vi "JSON to LVObject - Offset - Skipps Previous Data.vi"() -> ()   [LabVIEW 2017, in "JSON Serializable Serializer Tests.lvlib"]
uses:
  JSON Serializable Serializer Tests.lvlib
  JSON Serializable Serializer/JSON Serializable Serializer.lvclass
  Mock JSON Serializable/Mock JSON Serializable.lvclass/Mock JSON Serializable.ctl
  <vilib>/addons/_JKI Toolkits/Caraya/classes/Assert/Assert Equal Value and Type_Variant.vi
  <vilib>/addons/_JKI Toolkits/Caraya/classes/Test/Test.lvclass
  <vilib>/addons/_JKI Toolkits/Caraya/classes/Assert/Assert.lvclass
  Mock JSON Serializable/Mock JSON Serializable.lvclass
panel:
  out "error out":errorcluster
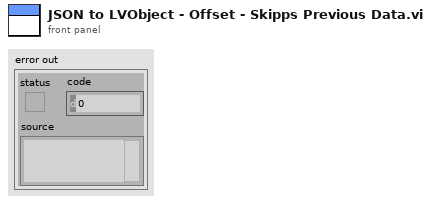
[diagram p1: front panel]
types:
  T1 = cluster{"LVClass Serializer":refnum<class "JSONtext LVClass Serializer.lvclass">, "<JSON>":string, "error in (no error)":errorcluster}
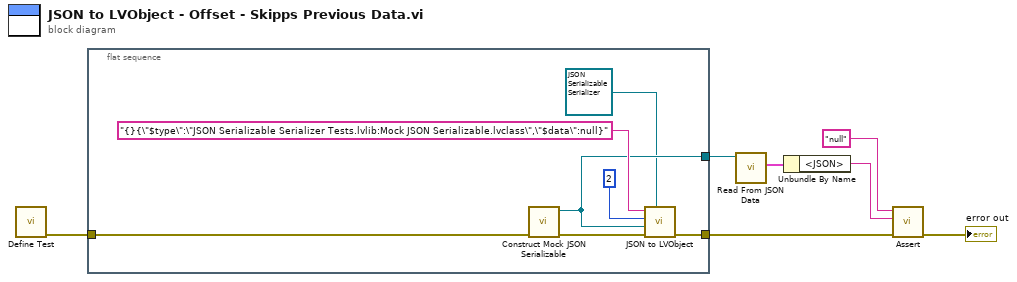
[diagram p0: block diagram]
diagram:
  n1 = call <vilib>:"Define Test.vi"() -> ("error out"=w7:errorcluster)  [unwired: 11 in]
  n2 = flat-sequence {
    tunnel: [w13] -> w5
    tunnel: w7 -> [w10]
    tunnel: [w9] -> w4
    frame #0 {
      n3 = call "Construct Mock JSON Serializable.vi"("error in (no error)"=w10) -> ("error out"=w11:errorcluster, "Mock JSON Serializable"=w9:refnum<class "Mock JSON Serializable.lvclass">)  [unwired: 9 in]
      n4 = call-dynamic "JSON to LVObject.vi"("JSON Serializable Serializer in"=refnum<class "JSON Serializable Serializer.lvclass"> refnum ("JSON Serializer.lvclass"), "error in (no error)"=w11, "Object Type"=w9, "Offset"=2, "JSON"="{}{\"$type\":\"JSON Serializable Serializer Tests.lvlib:Mock JSON Serializable.lvclass\",\"$data\":null}") -> ("error out"=w13:errorcluster)  [unwired: 5 in, 1 out]
    }
  }
  n5 = call "Read From JSON Data.vi"("Mock JSON Serializable in"=w4) -> ("From JSON Data"=w3:T1)  [unwired: 9 in, 1 out]
  n6 = Unbundle By Name(w3) -> ("<JSON>"=w2:string)
  n7 = call-poly <vilib>:"Assert.vi"("error in (no error)"=w5, "Y"=w2, "X"="null") -> ("error out"=→"error out":errorcluster)  [unwired: 8 in]
